vi "CHECK OUT ITEMS IN PGSQL.vi"(10 "USER/ITEM DATA TRANSFER":T1(array[cluster]), 11 "DATA IN":T2[](array[typedef])) -> ()   [LabVIEW 2019]
uses:
  Controls/Table Data Types/Inventory Data Type.ctl
  Controls/Column Names/Inventory Column Names.ctl
  <vilib>/addons/database/Connection.llb/DB Tools Open Connec (String).vi
  <vilib>/addons/database/NI_Database_API.lvlib
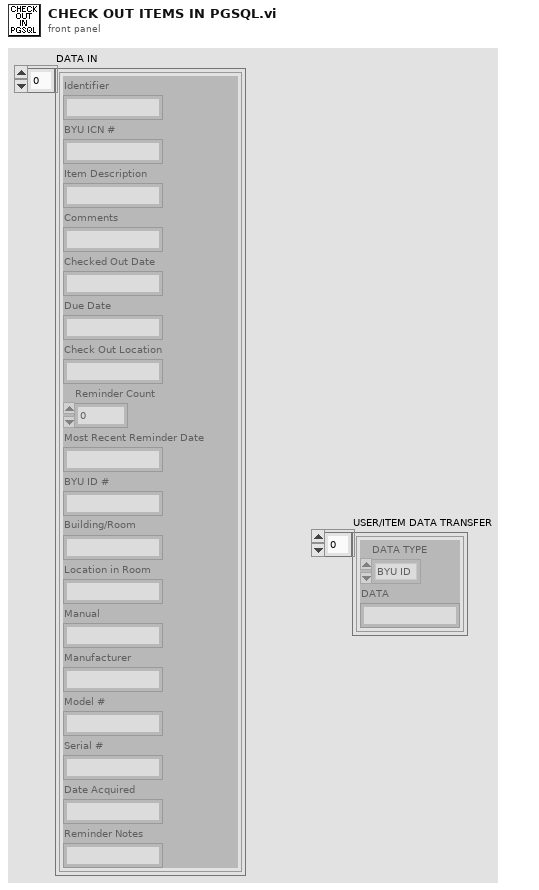
[diagram p1: front panel]
types:
  T1 = cluster{"DATA TYPE":enum16{"BYU ID", "ME#/IDENTIFIER", "BYU ICN"}, "DATA":string}[]
  T2 = typedef "Inventory Data Type.ctl" = cluster{"Identifier":string, "BYU ICN #":string, "Item Description":string, "Comments":string, "Checked Out Date":string, "Due Date":string, "Check Out Location":string, "Reminder Count":i32, "Most Recent Reminder Date":string, "BYU ID #":string, "Building/Room":string, "Location in Room":string, "Manual":string, "Manufacturer":string, "Model #":string, "Serial #":string, "Date Acquired":string, "Reminder Notes":string}
  T3 = cluster{"DATA TYPE":enum16{"BYU ID", "ME#/IDENTIFIER", "BYU ICN"}, "DATA":string}
  T4 = typedef "NI_Database_API.lvlib/Conn ObjectReference.ctl" = refnum<k1>
  T5 = typedef "Inventory Column Names.ctl" = string[]
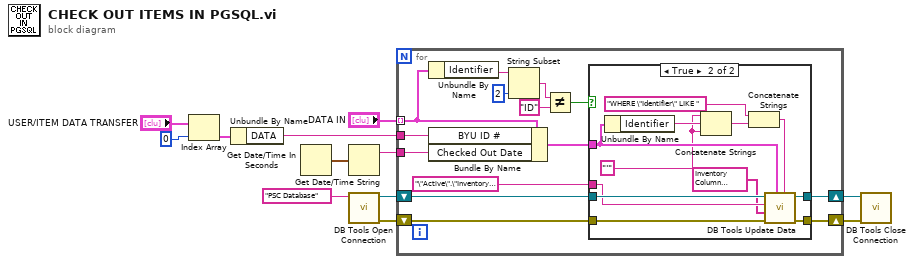
[diagram p0: block diagram]
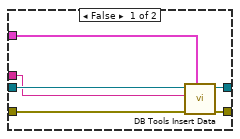
[diagram p2: hidden frame]
diagram:
  n1 = Index Array(array="USER/ITEM DATA TRANSFER", index=0) -> (element=w9:T3)
  n2 = Unbundle By Name(w9) -> ("DATA"=w8:string)
  n3 = Get Date/Time In Seconds() -> (seconds since 1Jan1904=w4:timestamp)
  n4 = Get Date/Time String(seconds (now)=w4) -> (date string=w3:string)  [unwired: 2 in, 1 out]
  n5 = call-poly <vilib>:"DB Tools Open Connection.vi"("connection information"="PSC Database") -> ("error out"=w5:errorcluster, "connection reference"=w6:T4)  [unwired: 7 in]
  n6 = for {
    tunnel: "DATA IN" -> [w22] mode=indexing
    tunnel: w8 -> [w17]
    shift-right: [w18] -> w1
    shift-left: w5 -> [w24]
    shift-right: [w19] -> w2
    shift-left: w6 -> [w25]
    tunnel: w3 -> [w21]
    n7 = Unbundle By Name(w22) -> ("Identifier"=w16:string)
    n8 = Bundle By Name(cluster=w22, "BYU ID #"=w17, "Checked Out Date"=w21) -> (w20:T2)
    n9 = String Subset(string=w16, length (rest)=2 ("length (rest)")) -> (substring=w14:string)  [unwired: 1 in]
    n10 = Not Equal?(x=w14, y="ID") -> (x != y?=w26:bool)
    n11 = case shown="True" w26 {
      tunnel: w25 -> [w32 w44]
      tunnel: w24 -> [w31 w43]
      tunnel: "\"Active\".\"Inventory\"" -> [w30 w42]
      tunnel: w20 -> [w29 w39]
      tunnel: [w28 w38] -> w19
      tunnel: [w27 w37] -> w18
      frame False {
        n12 = call <vilib>:"DB Tools Insert Data.vi"("data"=w29, "error in (no error)"=w31, "table"=w30, "connection reference"=w32) -> ("error out"=w27:errorcluster, "connection reference out"=w28:T4)  [unwired: 6 in]
      }
      frame True {
        w34 = "'"
        n13 = Unbundle By Name(w39) -> ("Identifier"=w35:string)
        n14 = Concatenate Strings(w34, w35, w34) -> (w36:string)
        n15 = Concatenate Strings("WHERE \"Identifier\" LIKE ", w36) -> (w40:string)
        n16 = call <vilib>:"DB Tools Update Data.vi"("condition"=w40, "data"=w39, "error in (no error)"=w43, "columns"=T5 ["\"Identifier\"", "\"BYU ICN #\"", "\"Item Description\"", "\"Comments\"", "\"Checked Out Date\"", "\"Due Date\"", "\"Check Out Location\"", "\"Reminder Count\"", "\"Most Recent Reminder Date\"", "\"BYU ID #\"", "\"Building/Room\"", "\"Location in Room\"", "\"Manual\"", "\"Manufacturer\"", "\"Model #\"", "\"Serial #\"", "\"Date Acquired\"", "\"Reminder Notes\""] ("INVENTORY COLUMN NAMES"), "table"=w42, "connection reference"=w44) -> ("error out"=w37:errorcluster, "connection reference out"=w38:T4)  [unwired: 4 in]
      }
    }
  }
  n17 = call <vilib>:"DB Tools Close Connection.vi"("error in (no error)"=w1, "connection reference"=w2) -> ()  [unwired: 5 in, 1 out]
